vi "经度.vi"(11 "经度":string) -> (1 "经度方向":string, 2 "经分":dbl, 3 "经度":i32)   [LabVIEW 2018]
panel:
  out "数字 3":i32
  out "数字 2":i32
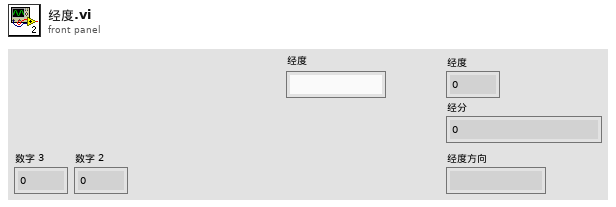
[diagram p1: front panel]
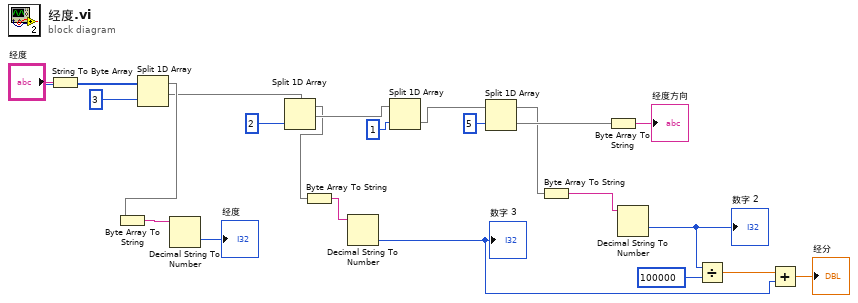
[diagram p0: block diagram]
diagram:
  n1 = String To Byte Array(string="经度") -> (unsigned byte array=w7:u8[])
  n2 = Split 1D Array(array=w7, index=3 ("索引")) -> (first subarray=w9:u8[], second subarray=w6:u8[])
  n3 = Byte Array To String(unsigned byte array=w9) -> (string=w11:string)
  n4 = Decimal String To Number(string=w11) -> (number=→"经度":i32)  [unwired: 2 in, 1 out]
  n5 = Split 1D Array(array=w6, index=2 ("索引")) -> (first subarray=w15:u8[], second subarray=w16:u8[])
  n6 = Byte Array To String(unsigned byte array=w15) -> (string=w14:string)
  n7 = Decimal String To Number(string=w14) -> (number=w22:i32)  [unwired: 2 in, 1 out]
  "数字 3" <- w22
  n8 = Split 1D Array(array=w16, index=1 ("索引")) -> (second subarray=w17:u8[])  [unwired: 1 out]
  n9 = Split 1D Array(array=w17, index=5 ("索引")) -> (first subarray=w18:u8[], second subarray=w19:u8[])
  n10 = Byte Array To String(unsigned byte array=w18) -> (string=w12:string)
  n11 = Byte Array To String(unsigned byte array=w19) -> (string=→"经度方向":string)
  n12 = Decimal String To Number(string=w12) -> (number=w20:i32)  [unwired: 2 in, 1 out]
  "数字 2" <- w20
  n13 = Divide(x=w20, y=100000) -> (x/y=w21:dbl)
  n14 = Add(x=w21, y=w22) -> (x+y=→"经分":dbl)
